vi "write out sonde row.vi"(0 "NI_report in":refnum<class "NI_report.lvclass">, 2 "Columns":i32[](array[numeric]), 3 "Column of Volume":i32, 5 "Sample Sheet Data Row Cluster":T1={"Head\nPressure"=0.0, "Depth"=0.0, "comment string"="", "Sonde Data Cluster"={"Cumulative\nVolume (ml)"=100.0, "Specific\nCond (mS)"=2.0, "Dissolved\nOxygen mg/L"=3.0, "pH"=4.0, "ORP"=5.0, "Temp\ndeg C"=26.0, "Salinity"=7.0}, "Aux1"=0.0, "Aux2"=0.0, "Aux3"=0.0} {"Sonde Data Cluster"."Salinity" format="%_3g"; "Sonde Data Cluster"."Temp\ndeg C" format="%_2g"; "Sonde Data Cluster"."ORP" format="%_4g"; "Sonde Data Cluster"."pH" format="%_4g"; "Sonde Data Cluster"."Dissolved\nOxygen mg/L" format="%_4g"; "Sonde Data Cluster"."Specific\nCond (mS)" format="%_4g"; "Sonde Data Cluster"."Cumulative\nVolume (ml)" format="%#_4g"}, 9 "row index":i32, 11 "error in (no error)":errorcluster, 13 "start of last occupied row":cluster{"row":i32, "column":i32}) -> (4 "NI_report out":refnum<class "NI_report.lvclass">, 14 "row index out":i32, 15 "error out":errorcluster)   [LabVIEW 2016]
uses:
  <vilib>/Utility/NIReport.llb/NI_report.lvclass
  sample data row cluster.ctl
  sonde cluster.ctl
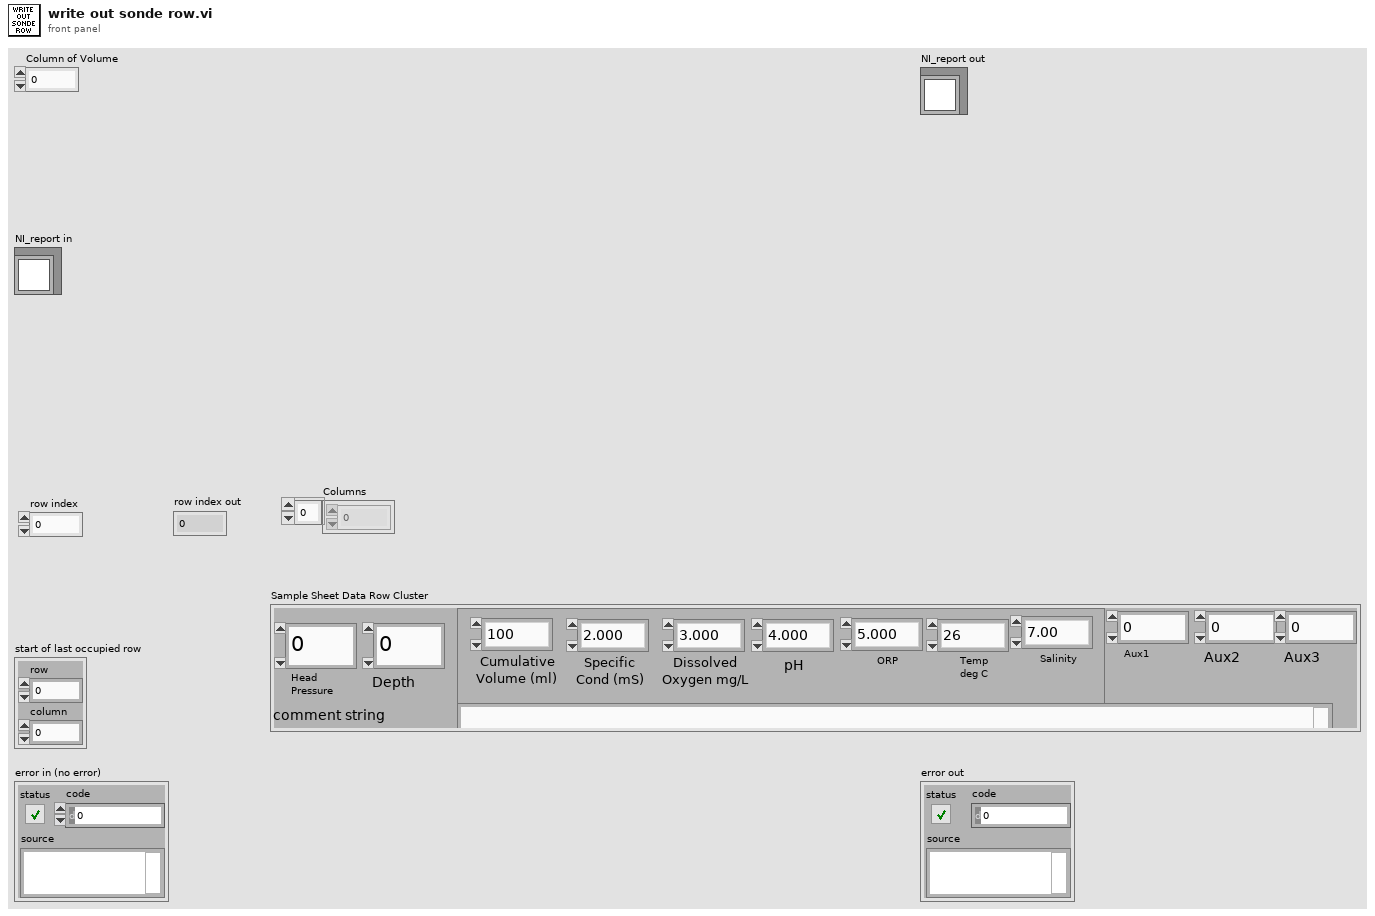
[diagram p1: front panel]
types:
  T1 = typedef "sample data row cluster.ctl" = cluster{"Head\nPressure":dbl, "Depth":dbl, "comment string":string, "Sonde Data Cluster":T2, "Aux1":dbl, "Aux2":dbl, "Aux3":dbl}
  T2 = typedef "sonde cluster.ctl" = cluster{"Cumulative\nVolume (ml)":dbl, "Specific\nCond (mS)":dbl, "Dissolved\nOxygen mg/L":dbl, "pH":dbl, "ORP":dbl, "Temp\ndeg C":dbl, "Salinity":dbl}
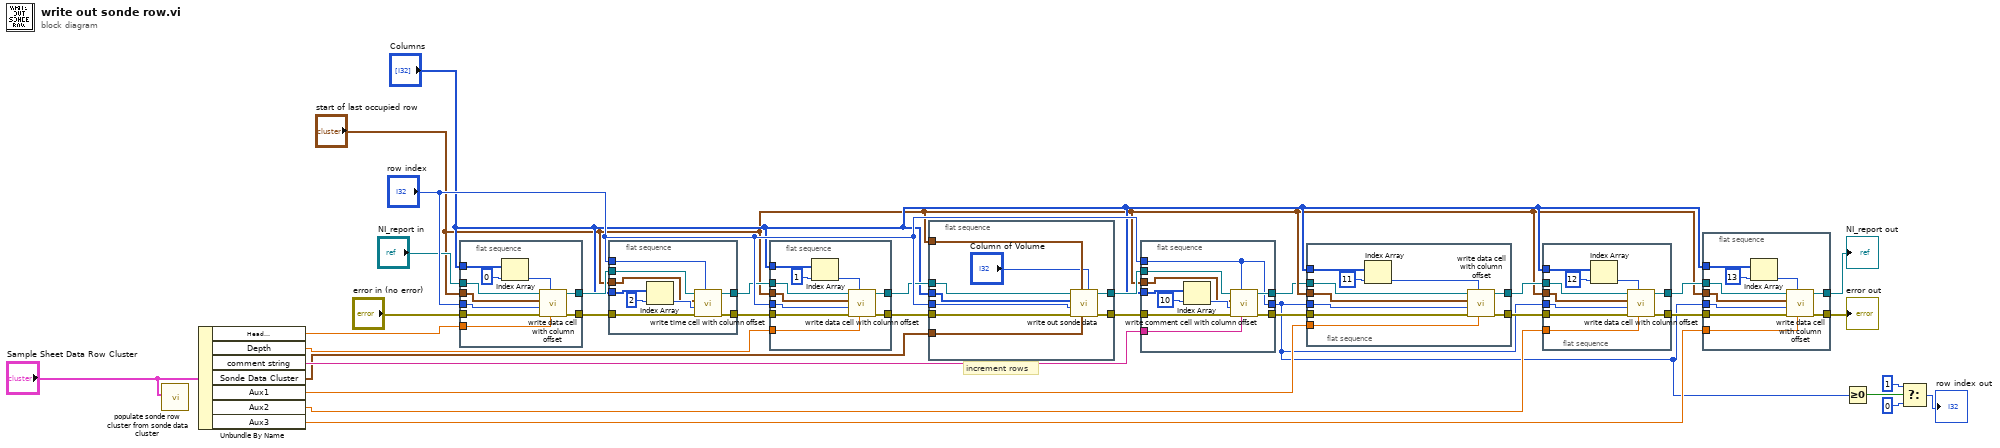
[diagram p0: block diagram]
diagram:
  # "increment rows"
  n1 = call "populate sonde row cluster from sonde data cluster.vi"("Sample Sheet Data Row Cluster"="Sample Sheet Data Row Cluster") -> ()  [unwired: 8 in, 3 out]
  n2 = Unbundle By Name("Sample Sheet Data Row Cluster") -> ("Head\nPressure"=w23:dbl, "Depth"=w22:dbl, "comment string"=w21:string, "Sonde Data Cluster"=w20:T2, "Aux1"=w14:dbl, "Aux2"=w3:dbl, "Aux3"=w2:dbl)
  n3 = flat-sequence {
    tunnel: "row index" -> [w44]
    tunnel: "start of last occupied row" -> [w43]
    tunnel: [w41] -> w30
    tunnel: [w40] -> w29
    tunnel: "NI_report in" -> [w38]
    tunnel: "error in (no error)" -> [w37]
    tunnel: "Columns" -> [w36]
    tunnel: w23 -> [w35]
    frame #0 {
      n4 = Index Array(array=w36, index=0) -> (element=w42:i32)
      n5 = call "write data cell with column offset.vi"("Data Input"=w35, "data column"=w42, "error in (no error)"=w37, "row offset"=w44, "start of last occupied row"=w43, "NI_report in"=w38) -> ("error out"=w41:errorcluster, "NI_report out"=w40:refnum<class "NI_report.lvclass">)  [unwired: 4 in]
    }
  }
  n6 = flat-sequence {
    tunnel: "row index" -> [w53]
    tunnel: "start of last occupied row" -> [w50]
    tunnel: w30 -> [w49]
    tunnel: w29 -> [w48]
    tunnel: [w47] -> w28
    tunnel: [w46] -> w27
    tunnel: "Columns" -> [w45]
    frame #0 {
      n7 = Index Array(array=w45, index=2) -> (element=w52:i32)
      n8 = call "write time cell with column offset.vi"("Header offset"=w53, "error in (no error)"=w49, "time column offset"=w52, "start of last occupied row"=w50, "NI_report in"=w48) -> ("error out"=w46:errorcluster, "NI_report out"=w47:refnum<class "NI_report.lvclass">)  [unwired: 5 in]
    }
  }
  n9 = flat-sequence {
    tunnel: "row index" -> [w63]
    tunnel: [w62] -> w33
    tunnel: "start of last occupied row" -> [w61]
    tunnel: w28 -> [w60]
    tunnel: w27 -> [w59]
    tunnel: [w58] -> w26
    tunnel: "Columns" -> [w57]
    tunnel: w22 -> [w54]
    frame #0 {
      n10 = Index Array(array=w57, index=1) -> (element=w55:i32)
      n11 = call "write data cell with column offset.vi"("Data Input"=w54, "data column"=w55, "error in (no error)"=w59, "row offset"=w63, "start of last occupied row"=w61, "NI_report in"=w60) -> ("error out"=w62:errorcluster, "NI_report out"=w58:refnum<class "NI_report.lvclass">)  [unwired: 4 in]
    }
  }
  n12 = flat-sequence {
    tunnel: "row index" -> [w72]
    tunnel: w33 -> [w71]
    tunnel: "Columns" -> [w70]
    tunnel: "start of last occupied row" -> [w69]
    tunnel: [w68] -> w32
    tunnel: [w67] -> w31
    tunnel: w26 -> [w66]
    tunnel: w20 -> [w64]
    frame #0 {
      n13 = call "write out sonde data.vi"("data column offset"="Column of Volume", "Sonde Data Cluster"=w64, "start of last occupied row"=w69, "error in (no error)"=w71, "Row Offset"=w72, "Header data columns"=w70, "NI_report in"=w66) -> ("error out"=w68:errorcluster, "NI_report out"=w67:refnum<class "NI_report.lvclass">)  [unwired: 3 in]
    }
  }
  n14 = flat-sequence {
    tunnel: "row index" -> [w73]
    tunnel: "Columns" -> [w80]
    tunnel: "start of last occupied row" -> [w79]
    tunnel: [w78] -> w5
    tunnel: w32 -> [w77]
    tunnel: [w76] -> w7
    tunnel: w31 -> [w75]
    tunnel: w21 -> [w74]
    tunnel: [w73] -> w1
    frame #0 {
      n15 = Index Array(array=w80, index=10) -> (element=w82:i32)
      n16 = call "write comment cell with column offset.vi"("comment string"=w74, "Row offset"=w73, "error in (no error)"=w77, "comment column offset"=w82, "start of last occupied row"=w79, "NI_report in"=w75) -> ("error out"=w78:errorcluster, "NI_report out"=w76:refnum<class "NI_report.lvclass">)  [unwired: 4 in]
    }
  }
  n17 = flat-sequence {
    tunnel: w1 -> [w92]
    tunnel: [w91] -> w12
    tunnel: "start of last occupied row" -> [w90]
    tunnel: w7 -> [w89]
    tunnel: w5 -> [w88]
    tunnel: [w87] -> w13
    tunnel: "Columns" -> [w86]
    tunnel: w14 -> [w83]
    frame #0 {
      n18 = Index Array(array=w86, index=11) -> (element=w84:i32)
      n19 = call "write data cell with column offset.vi"("Data Input"=w83, "data column"=w84, "error in (no error)"=w88, "row offset"=w92, "start of last occupied row"=w90, "NI_report in"=w89) -> ("error out"=w91:errorcluster, "NI_report out"=w87:refnum<class "NI_report.lvclass">)  [unwired: 4 in]
    }
  }
  n20 = flat-sequence {
    tunnel: w1 -> [w102]
    tunnel: [w101] -> w10
    tunnel: "start of last occupied row" -> [w100]
    tunnel: w13 -> [w99]
    tunnel: w12 -> [w98]
    tunnel: [w97] -> w11
    tunnel: "Columns" -> [w96]
    tunnel: w3 -> [w93]
    frame #0 {
      n21 = Index Array(array=w96, index=12) -> (element=w94:i32)
      n22 = call "write data cell with column offset.vi"("Data Input"=w93, "data column"=w94, "error in (no error)"=w98, "row offset"=w102, "start of last occupied row"=w100, "NI_report in"=w99) -> ("error out"=w101:errorcluster, "NI_report out"=w97:refnum<class "NI_report.lvclass">)  [unwired: 4 in]
    }
  }
  n23 = flat-sequence {
    tunnel: w1 -> [w112]
    tunnel: [w111] -> w4
    tunnel: "start of last occupied row" -> [w110]
    tunnel: w11 -> [w109]
    tunnel: w10 -> [w108]
    tunnel: [w107] -> w6
    tunnel: "Columns" -> [w106]
    tunnel: w2 -> [w103]
    frame #0 {
      n24 = Index Array(array=w106, index=13) -> (element=w104:i32)
      n25 = call "write data cell with column offset.vi"("Data Input"=w103, "data column"=w104, "error in (no error)"=w108, "row offset"=w112, "start of last occupied row"=w110, "NI_report in"=w109) -> ("error out"=w111:errorcluster, "NI_report out"=w107:refnum<class "NI_report.lvclass">)  [unwired: 4 in]
    }
  }
  n26 = Greater Or Equal To 0?(x=w1) -> (x >= 0?=w19:bool)
  n27 = Select(t=1, s=w19, f=0) -> (s? t:f=→"row index out":i32)
  "error out" <- w4
  "NI_report out" <- w6
